vi "Supply_Reset.vi"(8 "error in (no error)":errorcluster, 11 "SupplyControl in":refnum<class "SupplyControl.lvclass">) -> (0 "error out":errorcluster, 3 "SupplyControl out":refnum<class "SupplyControl.lvclass">)   [LabVIEW 2013, in "SupplyControl.lvclass"]
uses:
  SupplyControl.lvclass
  InstrControl.lvclass
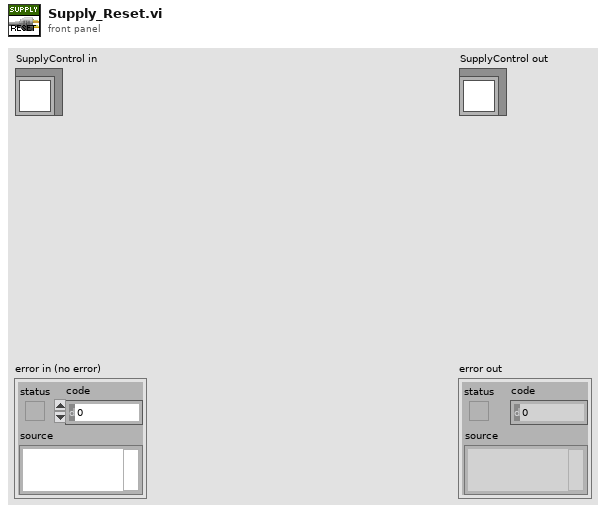
[diagram p1: front panel]
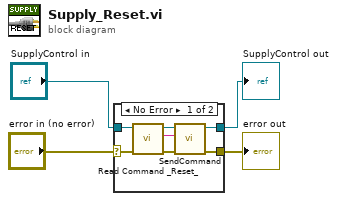
[diagram p0: block diagram]
diagram:
  n1 = case shown="No Error" "error in (no error)" {
    selector: "error in (no error)" -> [w6 w13]
    tunnel: [w7 w13] -> w3
    tunnel: [w8 w12] -> w1
    tunnel: "SupplyControl in" -> [w5 w12]
    frame No Error {
      n2 = call-dynamic "Read Command _Reset_.vi"("error in (no error)"=w6, "SupplyControl in"=w5) -> ("error out"=w9:errorcluster, "Command \"Reset\""=w10:string, "SupplyControl out"=w11:refnum<class "SupplyControl.lvclass">)  [unwired: 7 in]
      n3 = call "SendCommand.vi"("error in (no error)"=w9, "Command string"=w10, "InstControl in"=w11) -> ("error out"=w7:errorcluster, "InstControl out"=w8:refnum<class "SupplyControl.lvclass">)  [unwired: 7 in]
    }
    frame Error {
    }
  }
  "error out" <- w3
  "SupplyControl out" <- w1
